vi "Frequency Response Function (Real-Im) N-M.vi"(0 "time signals X":waveform(dbl)[](array[waveform]), 1 "restart averaging (F)":bool, 2 "window parameter":dbl=nan, 5 "time signals Y":waveform(dbl)[](array[waveform]), 7 "window":T1=1 items=["Rectangle"=0, "Hanning"=1, "Hamming"=2, "Blackman-Harris"=3, "Exact Blackman"=4, "Blackman"=5, "Flat Top"=6, "4 Term B-Harris "=7, "7 Term B-Harris"=8, "Low Sidelobe"=9, "Blackman Nuttall"=11, "Triangle"=30, "Bartlett-Hanning"=31, "Bohman"=32, "Parzen"=33, "Welch"=34, "Kaiser"=60, "Dolph-Chebyshev"=61, "Gaussian"=62], 11 "error in (no error)":errorcluster, 12 "averaging parameters":T2={"averaging mode"=enum."No averaging", "weighting mode"=enum."Exponential", "number of averages"=10} {"number of averages" min=1}, 13 "FRF Mode":enum16{"H1", "H2", "H3"}(ring), 14 "X-Y pairing":enum32{"ordered pairs", "all cross pairs"}(ring)) -> (3 "averaging done":bool, 4 "real parts":cluster{"f0":dbl, "df":dbl, "real part":dbl[]}[](array[cluster]) {"real part" format="%.2p"; "f0" format="%0.2p"; "df" format="%0.2p"}, 6 "imaginary parts":cluster{"f0":dbl, "df":dbl, "imag part":dbl[]}[](array[cluster]) {"imag part" format="%.2p"; "f0" format="%0.2p"; "df" format="%0.2p"}, 8 "coherences":cluster{"f0":dbl, "df":dbl, "coherence":dbl[]}[](array[cluster]) {"coherence" format="%.2g"; "df" format="%.2g"; "f0" format="%.2g"}, 10 "averages completed":dbl format="%.2p", 15 "error out":errorcluster)   [LabVIEW 2020, in "NI_MAPro.lvlib"]
doc: "Computes the frequency response and the coherence based on the input signals. Results are returned as <B>real part</B>, <B>imaginary part</B>, and <B>coherence</B>."
uses:
  NI_MAPro.lvlib
  windowTd.ctl
  2-chan State.ctl
  NI_AALPro.lvlib
  NI_MABase.lvlib
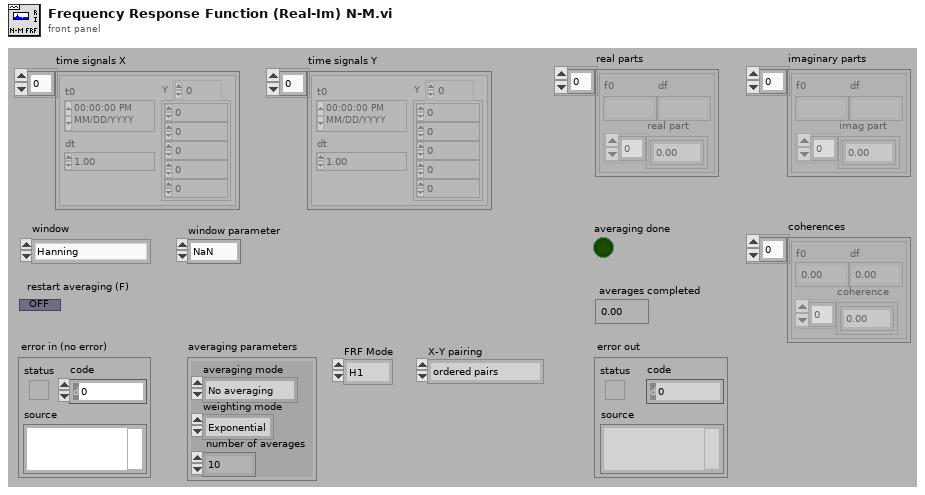
[diagram p1: front panel]
types:
  T1 = typedef "NI_AALPro.lvlib/windowTd.ctl" = u32
  T2 = cluster{"averaging mode":enum16{"No averaging", "Vector averaging", "RMS averaging", "Peak hold"}, "weighting mode":enum16{"Linear", "Exponential"}, "number of averages":u32}
  T3 = typedef "NI_MAPro.lvlib/2-chan State.ctl" = cluster{"Sx":cdb[], "Sy":cdb[], "Sxx":dbl[], "Syy":dbl[], "Sxy":cdb[], "block size":i32, "df":dbl, "dt":dbl, "avgs completed":dbl, "spectrum parameters":cluster{"averaging parameters":cluster{"averaging mode":enum16{"No averaging", "Vector averaging", "RMS averaging", "Peak hold"}, "weighting mode":enum16{"Linear", "Exponential"}, "number of averages":u32}, "window":T1}, "lin avg done":bool, "t0 history":dbl, "dt history":dbl, "timestamp":dbl}
  T4 = cluster{"f0":dbl, "df":dbl, "imag or phase":dbl[]}
  T5 = cluster{"f0":dbl, "df":dbl, "real or mag":dbl[]}[]
  T6 = cluster{"f0":dbl, "df":dbl, "imag or phase":dbl[]}[]
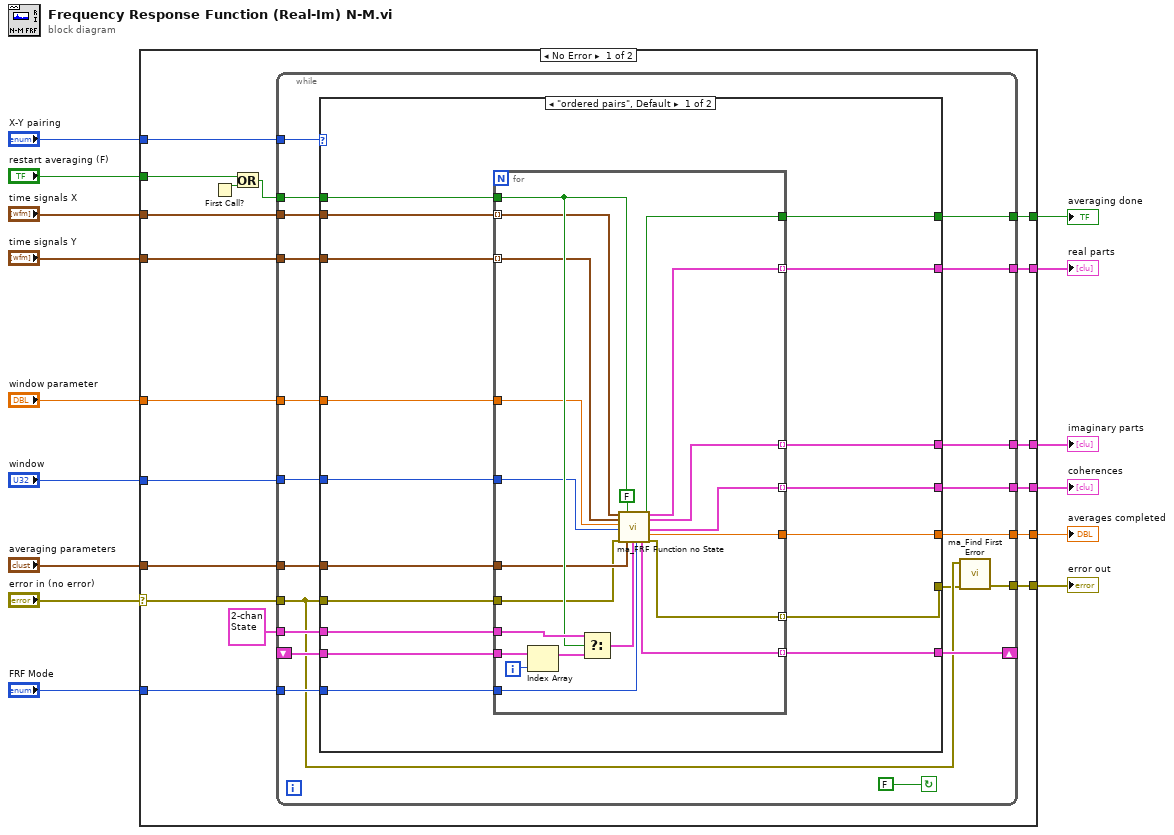
[diagram p0: block diagram]
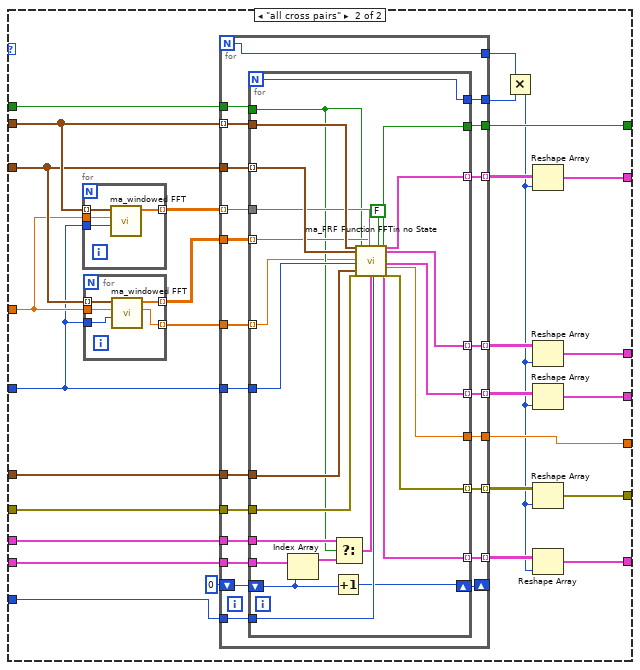
[diagram p2: hidden frame]
diagram:
  n1 = case shown="No Error" "error in (no error)" {
    selector: "error in (no error)" -> [w31 w178]
    tunnel: [w29 w178] -> w10
    tunnel: "FRF Mode" -> [w28 _]
    tunnel: "restart averaging (F)" -> [w27 _]
    tunnel: "time signals X" -> [w26 _]
    tunnel: "time signals Y" -> [w25 _]
    tunnel: "X-Y pairing" -> [w24 _]
    tunnel: "window" -> [w23 _]
    tunnel: "averaging parameters" -> [w22 _]
    tunnel: "window parameter" -> [w21 _]
    tunnel: [w20 _] -> w15
    tunnel: [w19 _] -> w14
    tunnel: [w18 _] -> w13
    tunnel: [w17 _] -> w12
    tunnel: [w16 _] -> w11
    frame No Error {
      n2 = First Call?() -> (First Call?: T/F=w33:bool)
      n3 = Or(x=w27, y=w33) -> (x .or. y?=w32:bool)
      n4 = while {
        tunnel: T3 {"Sx"=[], "Sy"=[], "Sxx"=[], "Syy"=[], "Sxy"=[], "block size"=0, "df"=0.0, "dt"=0.0, "avgs completed"=0.0, "spectrum parameters"={"averaging parameters"={"averaging mode"=enum."No averaging", "weighting mode"=enum."Linear", "number of averages"=0}, "window"=0}, "lin avg done"=FALSE, "t0 history"=0.0, "dt history"=0.0, "timestamp"=0.0} ("state info out") -> [w53]
        tunnel: w32 -> [w52]
        tunnel: w26 -> [w41]
        tunnel: w25 -> [w51]
        tunnel: w23 -> [w50]
        tunnel: w22 -> [w49]
        tunnel: w28 -> [w48]
        tunnel: [w47] -> w20
        tunnel: [w46] -> w16
        tunnel: w31 -> [w40]
        shift-right: [w44] -> _
        shift-left: _ -> [w43]
        tunnel: [w42] -> w29
        tunnel: [w39] -> w19
        tunnel: [w38] -> w18
        tunnel: [w37] -> w17
        tunnel: w24 -> [w35]
        tunnel: w21 -> [w34]
        stop <- FALSE continue-if-true
        n5 = case shown="\"ordered pairs\", Default" w35 {
          tunnel: w53 -> [w64 w120]
          tunnel: w52 -> [w70 w119]
          tunnel: w51 -> [w68 w97]
          tunnel: w50 -> [w67 w92]
          tunnel: w49 -> [w66 w118]
          tunnel: w48 -> [w62 w117]
          tunnel: [w55 w116] -> w47
          tunnel: [w59 w115] -> w46
          tunnel: [w61 w100] -> w44
          tunnel: w43 -> [w63 w114]
          tunnel: w41 -> [w69 w98]
          tunnel: w40 -> [w65 w113]
          tunnel: [w56 w109] -> w39
          tunnel: [w57 w106] -> w38
          tunnel: [w58 w105] -> w37
          tunnel: [w60 w103] -> w36
          tunnel: w34 -> [w54 w96]
          frame "ordered pairs", Default {
            n6 = for {
              tunnel: w70 -> [w84]
              tunnel: [w91] -> w55
              tunnel: [w90] -> w59
              tunnel: [w89] -> w56 mode=indexing
              tunnel: [w86] -> w57 mode=indexing
              tunnel: w64 -> [w85]
              tunnel: w69 -> [w83] mode=indexing
              tunnel: w68 -> [w77] mode=indexing
              tunnel: w67 -> [w82]
              tunnel: w66 -> [w81]
              tunnel: w62 -> [w80]
              tunnel: [w79] -> w58 mode=indexing
              tunnel: w65 -> [w78]
              tunnel: [w76] -> w61 mode=indexing
              tunnel: w63 -> [w74]
              tunnel: [w72] -> w60 mode=indexing
              tunnel: w54 -> [w71]
              i -> [w75]
              n7 = Index Array(array=w74, index=w75) -> (element=w73:T3)
              n8 = Select(t=w85, s=w84, f=w73) -> (s? t:f=w88:T3)
              n9 = call "ma_FRF Function no State.vi"("time signal X"=w83, "time signal Y"=w77, "window parameter"=w71, "window"=w82, "error in (no error)"=w78, "restart averaging (F)"=w84, "averaging parameters"=w81, "mag-phase"=FALSE, "state info"=w88, "FRF Mode"=w80) -> ("averaging done"=w91:bool, "state info out"=w76:T3, "real or mag"=w89:cluster{"f0":dbl, "df":dbl, "real or mag":dbl[]}, "imag or phase"=w86:T4, "coherence"=w79:cluster{"f0":dbl, "df":dbl, "coherence":dbl[]}, "averages completed"=w90:dbl, "error out"=w72:errorcluster)  [unwired: 1 in, 2 out]
            }
          }
          frame "all cross pairs" {
            n10 = for {
              tunnel: w98 -> [w129] mode=indexing
              tunnel: [w128] -> w95 mode=indexing
              tunnel: w96 -> [w127]
              tunnel: w92 -> [w126]
              n11 = call "ma_windowed FFT.vi"("window"=w126, "window parameter"=w127, "time signal X"=w129) -> ("Sx"=w128:cdb[])  [unwired: 6 in, 2 out]
            }
            n12 = for {
              tunnel: w97 -> [w125] mode=indexing
              tunnel: [w124] -> w94 mode=indexing
              tunnel: w96 -> [w123]
              tunnel: [w122] -> w93 mode=indexing
              tunnel: w92 -> [w121]
              n13 = call "ma_windowed FFT.vi"("window"=w121, "window parameter"=w123, "time signal X"=w125) -> ("df"=w122:dbl, "Sx"=w124:cdb[])  [unwired: 6 in, 1 out]
            }
            n14 = for {
              N -> [w137]
              tunnel: w120 -> [w152]
              tunnel: w119 -> [w151]
              tunnel: w97 -> [w150]
              tunnel: w92 -> [w149]
              tunnel: w118 -> [w148]
              tunnel: w117 -> [w147]
              tunnel: [w146] -> w116
              tunnel: [w145] -> w115
              tunnel: [w144] -> w102 mode=indexing
              tunnel: w114 -> [w143]
              tunnel: w98 -> [w142] mode=indexing
              tunnel: w113 -> [w141]
              tunnel: [w140] -> w112 mode=indexing
              tunnel: [w139] -> w108 mode=indexing
              tunnel: [w138] -> w107 mode=indexing
              tunnel: [w137] -> w111
              tunnel: [w136] -> w110
              tunnel: [w135] -> w104 mode=indexing
              shift-right: [w133] -> _
              shift-left: 0 -> [w134]
              tunnel: w95 -> [w132] mode=indexing
              tunnel: w94 -> [w131]
              tunnel: w93 -> [w130]
              n15 = for {
                N -> [w161]
                tunnel: w151 -> [w155]
                tunnel: [w158] -> w146
                tunnel: [w177] -> w145
                tunnel: w152 -> [w174]
                tunnel: w142 -> [w173]
                tunnel: w150 -> [w169] mode=indexing
                tunnel: w149 -> [w165]
                tunnel: w148 -> [w172]
                tunnel: w147 -> [w171]
                tunnel: w141 -> [w170]
                tunnel: [w153] -> w144 mode=indexing
                tunnel: w143 -> [w168]
                tunnel: [w166] -> w135 mode=indexing
                tunnel: [w164] -> w140 mode=indexing
                tunnel: [w163] -> w139 mode=indexing
                tunnel: [w162] -> w138 mode=indexing
                tunnel: [w161] -> w136
                shift-right: [w159] -> w133
                shift-left: w134 -> [w160]
                tunnel: w132 -> [w157]
                tunnel: w131 -> [w156] mode=indexing
                tunnel: w130 -> [w154] mode=indexing
                n16 = Index Array(array=w168, index=w160) -> (element=w167:T3)
                n17 = Increment(x=w160) -> (x+1=w159:i32)
                n18 = Select(t=w174, s=w155, f=w167) -> (s? t:f=w176:T3)
                n19 = call "ma_FRF Function FFTin no State.vi"("time signal X"=w173, "time signal Y"=w169, "df"=w154, "window"=w165, "error in (no error)"=w170, "restart averaging (F)"=w155, "averaging parameters"=w172, "mag-phase"=FALSE, "Sy"=w156, "state info"=w176, "Sx"=w157, "FRF Mode"=w171) -> ("averaging done"=w158:bool, "state info out"=w153:T3, "real or mag"=w164:cluster{"f0":dbl, "df":dbl, "real or mag":dbl[]}, "imag or phase"=w163:T4, "coherence"=w162:cluster{"f0":dbl, "df":dbl, "coherence":dbl[]}, "averages completed"=w177:dbl, "error out"=w166:errorcluster)  [unwired: 9 in]
              }
            }
            n20 = Multiply(x=w111, y=w110) -> (x*y=w101:i32)
            n21 = Reshape Array(w112, w101) -> (w109:T5)
            n22 = Reshape Array(w108, w101) -> (w106:T6)
            n23 = Reshape Array(w107, w101) -> (w105:cluster{"f0":dbl, "df":dbl, "coherence":dbl[]}[])
            n24 = Reshape Array(w104, w101) -> (w103:errorcluster[])
            n25 = Reshape Array(w102, w101) -> (w100:T3[])
          }
        }
        n26 = call "ma_Find First Error.vi"("error array in"=w36, "error in 1 (no error)"=w40) -> ("error out"=w42:errorcluster)  [unwired: 2 in, 3 out]
      }
    }
    frame Error {
    }
  }
  "error out" <- w10
  "averages completed" <- w11
  "averaging done" <- w15
  "coherences" <- w12
  "real parts" <- w14
  "imaginary parts" <- w13
